vi "Scale Object.vi"(8 "error in (no error)":errorcluster, 10 "Scale":cluster{"X":sgl, "Y":sgl, "Z":sgl}, 11 "Scene.Object In":refnum<vi>) -> (0 "error out":errorcluster, 3 "Scene.Object Out":refnum<vi>)   [LabVIEW 2017, in "NI_3D Picture Control.lvlib"]
doc: "Uniformly scales an object in a 3D scene by the factors you specify. This VI performs a relative scale from the object's current position."
uses:
  <vilib>/picture/3D Picture Control/NI_3D Picture Control.lvlib
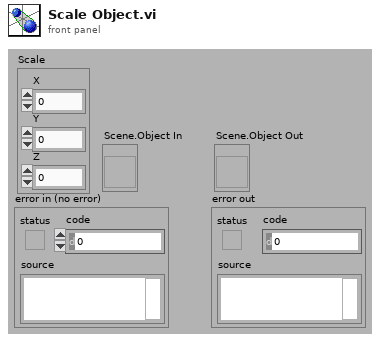
[diagram p1: front panel]
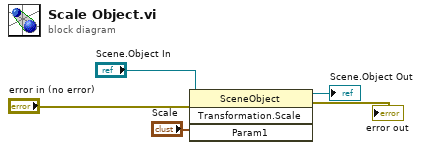
[diagram p0: block diagram]
diagram:
  n1 = invoke class="SceneObject" method="Transformation.Scale"(reference="Scene.Object In", error in="error in (no error)", "Param1"="Scale") -> (reference out=→"Scene.Object Out":refnum<vi>, error out=→"error out":errorcluster)  [unwired: 1 in, 2 out]
